vi "Cleanup Session.vi"(8 "error in":errorcluster, 11 "Plugin in":refnum<class "MP710995.lvclass">) -> (0 "error out":errorcluster, 3 "Plugin out":refnum<class "MP710995.lvclass">)   [LabVIEW 2025, in "MP710995.lvlib" / "MP710995.lvclass"]
uses:
  MP710995.lvclass
  MP710995.lvclass/MP710995.ctl
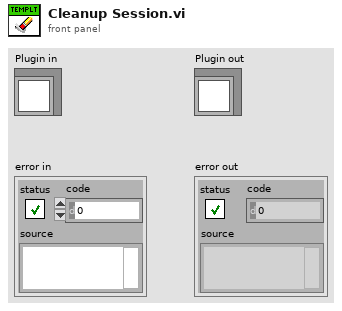
[diagram p1: front panel]
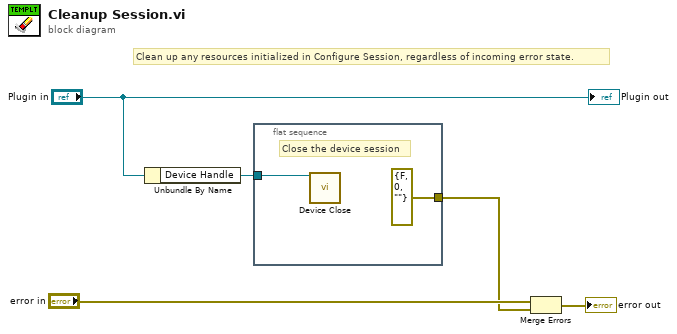
[diagram p0: block diagram]
diagram:
  # "Clean up any resources initialized in Configure Session, regardless of incoming error state."
  n1 = Unbundle By Name("Plugin in") -> ("Device Handle"=w2:refnum<visa-resource-name>)
  n2 = flat-sequence {
    tunnel: w2 -> [w6]
    tunnel: [errorcluster {"status"=FALSE, "code"=0, "source"=""} ("error in")] -> w1
    frame #0 {
      # "Close the device session"
      n3 = call "Device Close.vi"("VISA Rresource Name"=w6) -> ()  [unwired: 14 in, 1 out]
    }
  }
  n4 = Merge Errors("error in", w1) -> (→"error out":errorcluster)
  "Plugin out" <- "Plugin in"
